vi "getScannerConfig.vi"(8 "Error In":errorcluster, 11 "Config File Path":path) -> (0 "Error Out":errorcluster, 3 "comPort":string)   [LabVIEW 2018]
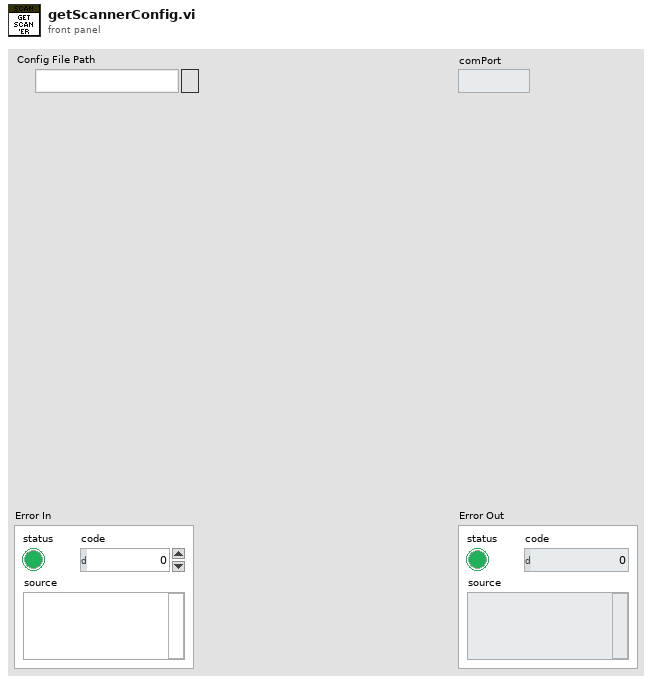
[diagram p1: front panel]
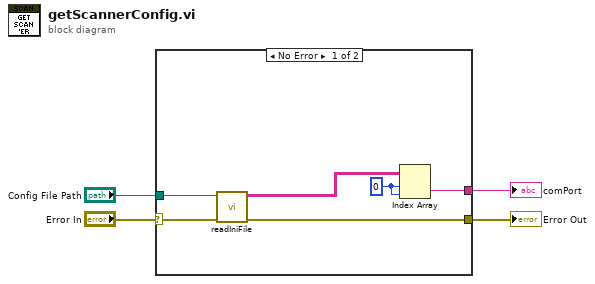
[diagram p0: block diagram]
diagram:
  n1 = case shown="No Error" "Error In" {
    selector: "Error In" -> [w10 w11]
    tunnel: [w9 w11] -> w1
    tunnel: "Config File Path" -> [w8 _]
    tunnel: [w5 _] -> w2
    frame No Error {
      w6 = 0 ("index (row)")
      n2 = call "readIniFile.vi"("Error In"=w10, "File Path Control"=w8) -> ("Error Out"=w9:errorcluster, "Value"=w7:string[][])  [unwired: 8 in]
      n3 = Index Array(array=w7, index (row)=w6, index (col)=w6) -> (element=w5:string)
    }
    frame Error {
    }
  }
  "Error Out" <- w1
  "comPort" <- w2
